vi "Evaluate.vi"(8 "error in (no error)":errorcluster, 10 "Data":refnum<class "Data.lvclass">[](array[class]), 11 "Test Double Data Tracker in":refnum<class "Test Double Data Tracker.lvclass">) -> (0 "error out":errorcluster, 3 "Tracker Data":refnum<class "Tracker Data.lvclass">)   [LabVIEW 2020, in "Test.lvlib" / "Test Double Data Tracker.lvclass"]
doc: "Evaluate the tracked Data and return Tracker Data.\n\nThe parent implementation does nothing."
uses:
  Test Double Data Tracker.lvclass
  PPL/HDH.Data.Generic.lvlibp/Data.lvclass
  PPL/HDH.Actor Framework.Core.Data Tracker.lvlibp/Data Tracker/Data/Tracker Data.lvclass
  PPL/HDH.Actor Framework.Core.Data Tracker.lvlibp/Messages for this Actor/Data Tracker Msg/Data Tracker Msg.lvclass
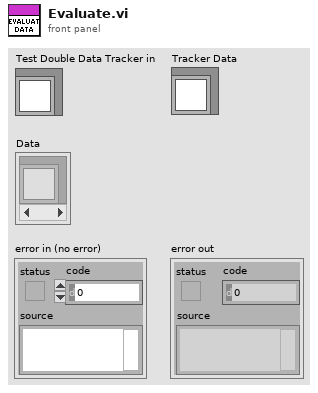
[diagram p1: front panel]
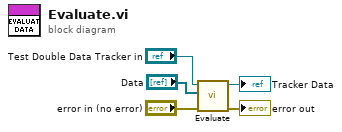
[diagram p0: block diagram]
diagram:
  n1 = call-parent "Evaluate.vi"("error in (no error)"="error in (no error)", "Data"="Data", "Data Tracker Msg in"="Test Double Data Tracker in") -> ("error out"=→"error out":errorcluster, "Tracker Data"=→"Tracker Data":refnum<class "Tracker Data.lvclass">)  [unwired: 7 in]
